vi "Robot Main.vi"() -> ()   [LabVIEW 2014]
doc: "This VI implements the framework and scheduler for your robotics program. It should not be necessary to modify the framework. You are expected to add your code to the VIs called from Robot Main - the ones located in the Team Code folder within the project."
uses:
  Robot Global Data.vi
panel:
  out "Waveform Chart":T1(graph)
  in  "Finish":bool
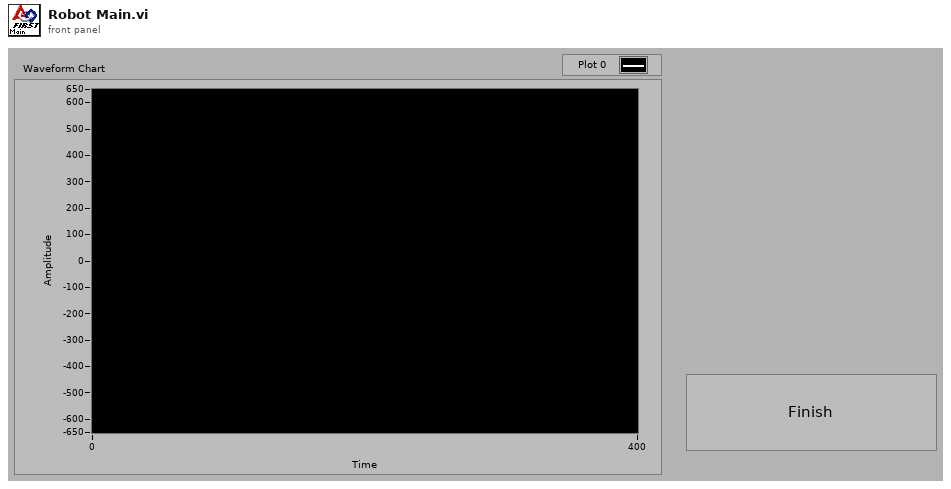
[diagram p1: front panel]
types:
  T1 = cluster{"LeftOutput":dbl, "LeftVelocity":dbl, "RightOutput":dbl, "RightVelocity":dbl}
  T2 = typedef "WPI_DriverStationMatch Info.ctl" = cluster{"Autonomous Elapsed Seconds":dbl, "TeleOp Elapsed Seconds":dbl, "Disabled Elapsed Seconds":dbl, "Visited Autonomous":bool, "Visited TeleOp":bool, "Visited Disabled":bool, "Autonomous Settings":cluster{"Autonomous Style":enum16{"Iterative", "Independent"}, "VI Refnum":refnum<vi>}}
  T3 = typedef "WPI_DriverStationDerivedRobotMode.ctl" = enum16{"Init", "Execute", "Stop"}
  T4 = enum16{"Autonomous Disabled", "Autonomous Enabled", "Teleop Disabled", "Teleop Enabled", "Disconnected", "Finish", "Test Disabled", "Test Enabled"}
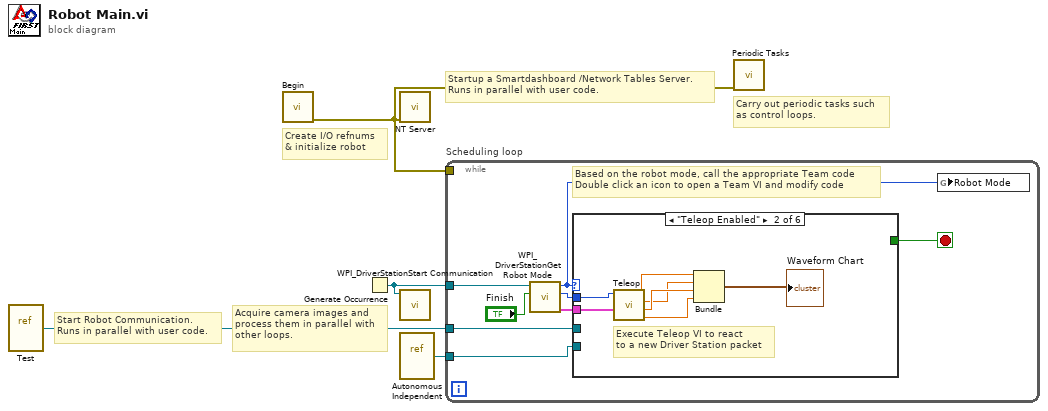
[diagram p0: block diagram]
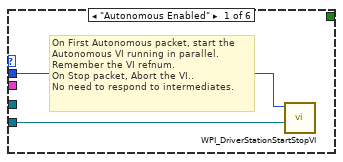
[diagram p2: hidden frame]
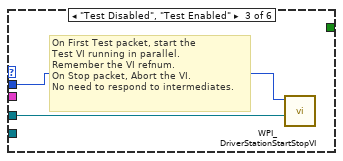
[diagram p3: hidden frame]
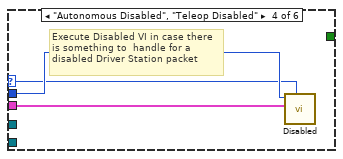
[diagram p4: hidden frame]
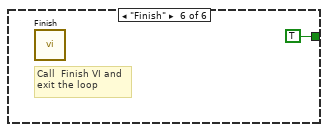
[diagram p6: hidden frame]
diagram:
  # "Startup a Smartdashboard /Network Tables Server.\nRuns in parallel with user code."
  # "Carry out periodic tasks such\nas control loops."
  # "Acquire camera images and\nprocess them in parallel with\nother loops."
  # "Create I/O refnums\n& initialize robot"
  # "Start Robot Communication.\nRuns in parallel with user code."
  n1 = vi-ref "Test.vi"() -> (w2:refnum<vi>)
  n2 = call "Begin.vi"() -> ("error out"=w1:errorcluster)  [unwired: 1 in, 10 out]
  n3 = Generate Occurrence() -> (w4:refnum<k4>)
  n4 = call <vilib>:"NT Server.vi"("error in (no error)"=w1) -> ()  [unwired: 11 in]
  n5 = call <vilib>:"WPI_DriverStationStart Communication.vi"("occurrence"=w4) -> ()  [unwired: 1 in, 10 out]
  n6 = vi-ref "Autonomous Independent.vi"() -> (w3:refnum<vi>)
  n7 = while "Scheduling loop" {
    tunnel: w4 -> [w11]
    tunnel: w1 -> [_]
    tunnel: w3 -> [w7]
    tunnel: w2 -> [w6]
    stop <- w8 stop-if-true
    # "Based on the robot mode, call the appropriate Team code\nDouble click an icon to open a Team VI and modify code"
    n8 = call <vilib>:"WPI_DriverStationGet Robot Mode.vi"("Finish"="Finish", "DS Occurrence"=w11) -> ("Match Info out"=w9:T2, "Call Context"=w12:T3, "Robot Mode"=w5:T4)  [unwired: 7 out]
    n9 = case shown="\"Teleop Enabled\"" w5 {
      selector: w5 -> [_ _ _ w24 _ _]
      tunnel: w12 -> [w14 w21 w23 w26 _ _]
      tunnel: w9 -> [_ w20 _ w25 _ _]
      tunnel: [_ _ _ _ _ TRUE] -> w8
      tunnel: w7 -> [w13 _ _ _ _ _]
      tunnel: w6 -> [_ _ w22 _ _ _]
      frame "Autonomous Enabled" {
        # "On First Autonomous packet, start the\nAutonomous VI running in parallel.\nRemember the VI refnum.\nOn Stop packet, Abort the VI..\nNo need to respond to intermediates."
        n10 = call <vilib>:"WPI_DriverStationStartStopVI.vi"("VI in"=w13, "Call Context"=w14) -> ()  [unwired: 10 in]
      }
      frame "Teleop Enabled" {
        # "Execute Teleop VI to react\nto a new Driver Station packet"
        n11 = call "Teleop.vi"("Match Info"=w20, "Call Context"=w21) -> ("RightVelocity"=w19:dbl, "RightOutput"=w18:dbl, "LeftVelocity"=w17:dbl, "LeftOutput"=w16:dbl)  [unwired: 1 in, 5 out]
        n12 = Bundle("LeftOutput"=w16, "LeftVelocity"=w17, "RightOutput"=w18, "RightVelocity"=w19) -> (→"Waveform Chart":T1)  [unwired: 1 in]
      }
      frame "Test Disabled", "Test Enabled" {
        # "On First Test packet, start the\nTest VI running in parallel.\nRemember the VI refnum.\nOn Stop packet, Abort the VI.\nNo need to respond to intermediates."
        n13 = call <vilib>:"WPI_DriverStationStartStopVI.vi"("VI in"=w22, "Call Context"=w23) -> ()  [unwired: 10 in]
      }
      frame "Autonomous Disabled", "Teleop Disabled" {
        # "Execute Disabled VI in case there\nis something to  handle for a\ndisabled Driver Station packet"
        n14 = call "Disabled.vi"("Robot Mode"=w24, "Match Info"=w25, "Call Context"=w26) -> ()  [unwired: 1 in, 8 out]
      }
      frame "Disconnected" {
        # "Driver Station packet didn't arrive.\nPossibly useful for diagnostics"
      }
      frame "Finish" {
        # "Call  Finish VI and\nexit the loop"
        n15 = call "Finish.vi"() -> ()  [unwired: 1 in, 7 out]
      }
    }
    n16 = global write "Robot Global Data.vi" "Robot Mode"(w5) -> ()
  }
  n17 = call "Periodic Tasks.vi"("error in"=w1) -> ()  [unwired: 1 in, 10 out]
